vi "Get Histogram.vi"(0 "DeviceIndex":i32) -> (2 "Histograms":u32[][](graph), 3 "IntegralCount":i32[](array[numeric]), 4 "Overflow":bool)   [LabVIEW 2011]
uses:
  MT Scan/SubVIs/hhlib.dll
panel:
  out "Flags":i32 format="%.0b"
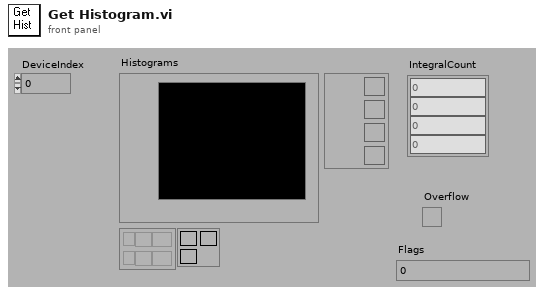
[diagram p1: front panel]
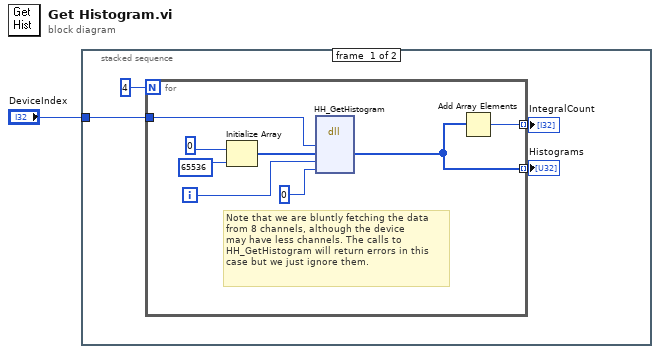
[diagram p0: block diagram]
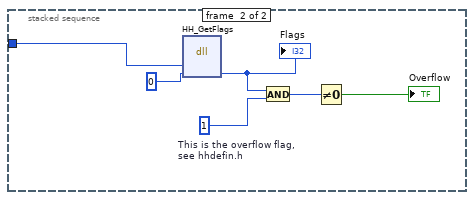
[diagram p2: hidden frame]
diagram:
  n1 = stacked-sequence {
    tunnel: "DeviceIndex" -> [w2 w16]
    frame #0 {
      n2 = for {
        N: 4 -> [_]
        tunnel: [w11] -> w3 mode=indexing
        tunnel: [w6] -> w4 mode=indexing
        tunnel: w2 -> [w8]
        i -> [w9]
        # "Note that we are bluntly fetching the data \nfrom 8 channels, although the device \nmay have less channels. The calls to\nHH_GetHistogram will return errors in this \ncase but we just ignore them."
        n3 = Initialize Array "Initialize Array"(u32 0, 65536) -> (w10:u32[])
        n4 = dll-call lib="C:/Users/Core-FCS/Desktop/AbelFCS/MT Scan/SubVIs/hhlib.dll" fn="HH_GetHistogram"("devidx"=w8, "Chcount"=w10, "channel"=w9, "clear"=0) -> ("Chcount"=w6:u32[])  [unwired: 7 in, 2 out]
        n5 = Add Array Elements(numeric array=w6) -> (sum=w11:u32)
      }
      "Histograms" <- w4
      "IntegralCount" <- w3
    }
    frame #1 {
      w18 = 1  # This is the overflow flag,  see hhdefin.h
      n6 = dll-call lib="C:/Users/Core-FCS/Desktop/AbelFCS/MT Scan/SubVIs/hhlib.dll" fn="HH_GetFlags"("devidx"=w16, "flags"=0) -> ("flags"=w14:i32)  [unwired: 5 in, 2 out]
      "Flags" <- w14
      n7 = And(x=w14, y=w18) -> (x .and. y?=w15:i32)
      n8 = Not Equal To 0?(x=w15) -> (x != 0?=→"Overflow":bool)
    }
  }
